vi "captPT01.vi"(6 "Graph in 2":cluster{dbl[], dbl[]}, 8 "error in":errorcluster, 9 "Length 2":i32=250, 11 "ON 2":bool) -> (0 "error out 2":errorcluster caption="error out", 2 "Values 2":cluster{dbl[], dbl[]})   [LabVIEW 2012]
uses:
  GlobalVariables/GantnerParameters.vi
  GlobalVariables/ZeroTimeGraph.vi
  GlobalVariables/CommunicationActivity.vi
  ISMBUS32.DLL
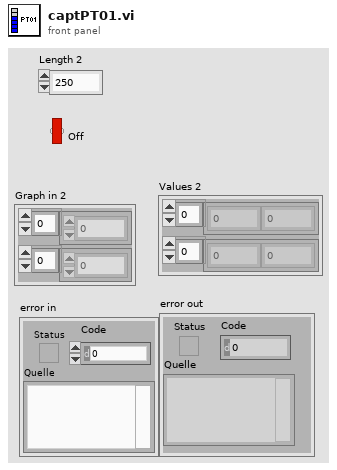
[diagram p1: front panel]
types:
  T1 = typedef "ISMBUS_Module.ctl" = cluster{"ModuleAddress":i32, "ModuleKindIndex":i32, "ModuleKind":string, " Protocol":string, " BaudRate":i32, "CharFormat":string, "BaudRateIndex":i32, "FormatIndex":i32, "ProtocolIndex":i32, "Location":string, "SerialNumber":string, "Vendor":string, "HWRelease":string, "SWRelease":string, "ControllerType":string, "ChannelList":T2[], "ChannelCount":i32, " COM Port":i32}
  T2 = typedef "ISMBUS_Channel.ctl" = cluster{" Description":string, " ChannelKindIndex":i32, "ChannelFormatIndex":i32, " FieldLength":i32, "Precision":i32, "Unit":string, "Mode":i32}
  T3 = cluster{"Module":T1, "PT01 chanel":u32, "Temperature chanel":u32, "HEV01 chanel":u32, "HEV02 chanel":u32, "PressureLimit":dbl}
  T4 = cluster{"KellerActive":bool, "GantnerActive":bool, "BrooksActive":bool}
  T5 = cluster{"KellerActive":bool, bool, "BrooksActive":bool}
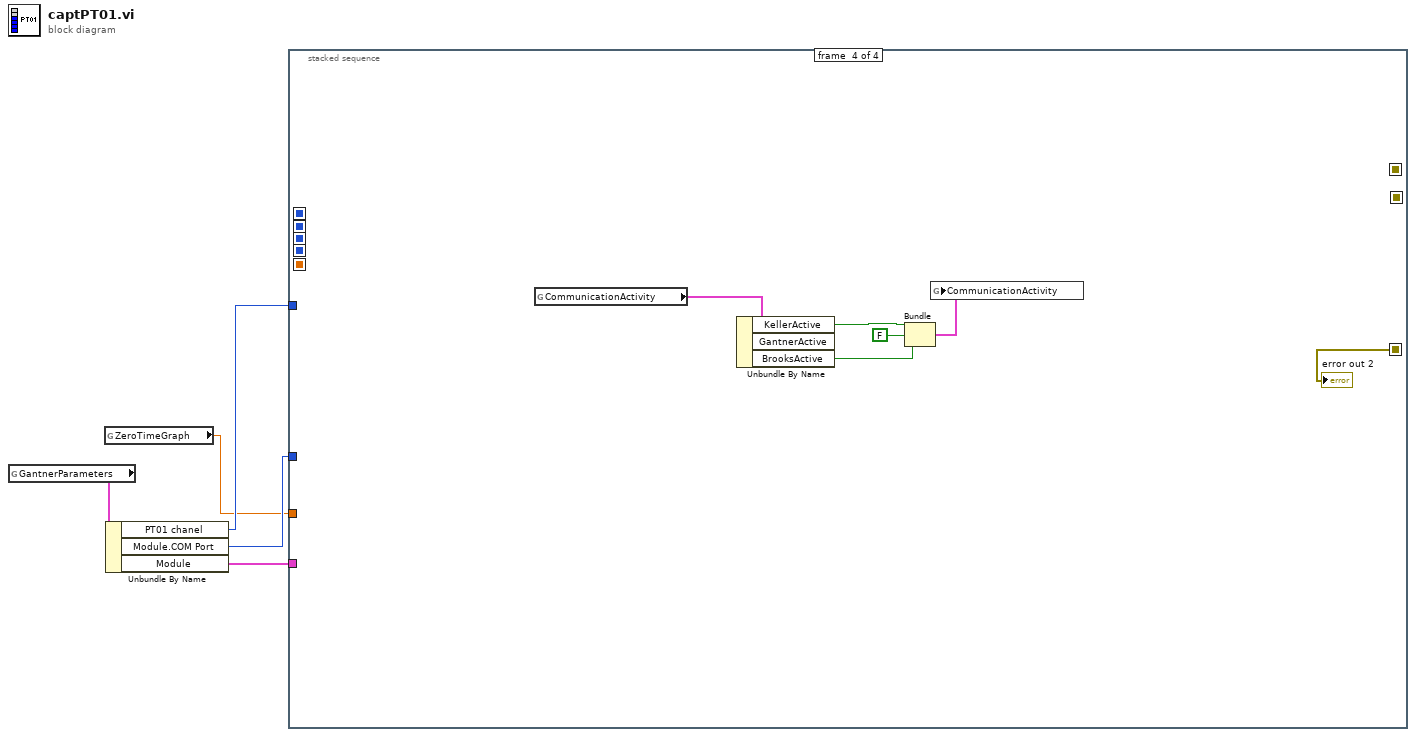
[diagram p0: block diagram]
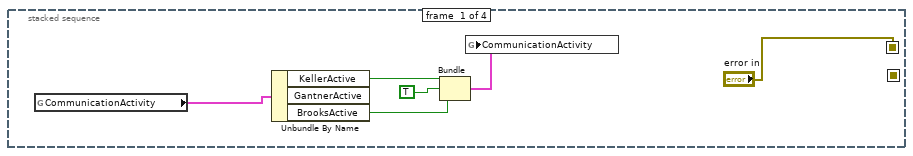
[diagram p2: hidden frame]
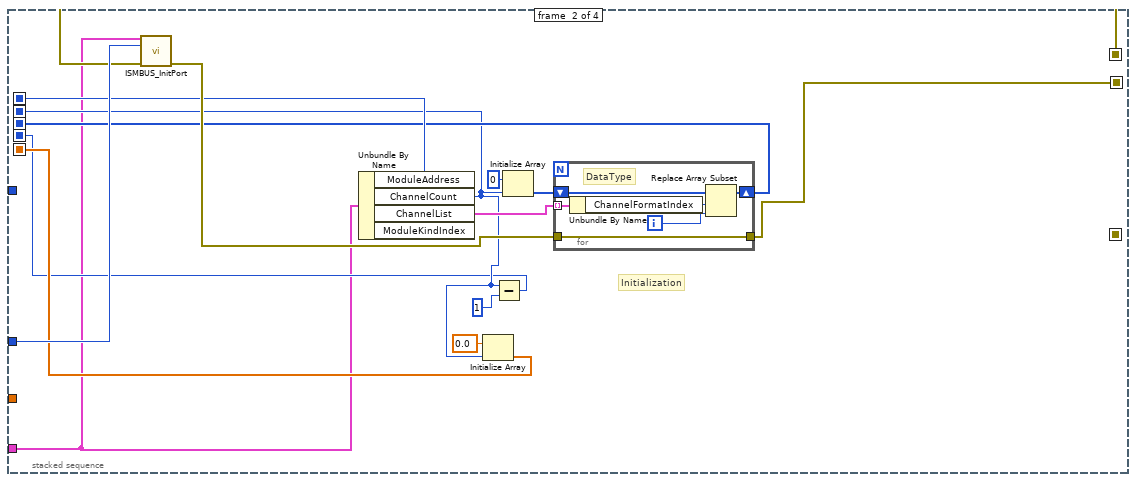
[diagram p3: hidden frame]
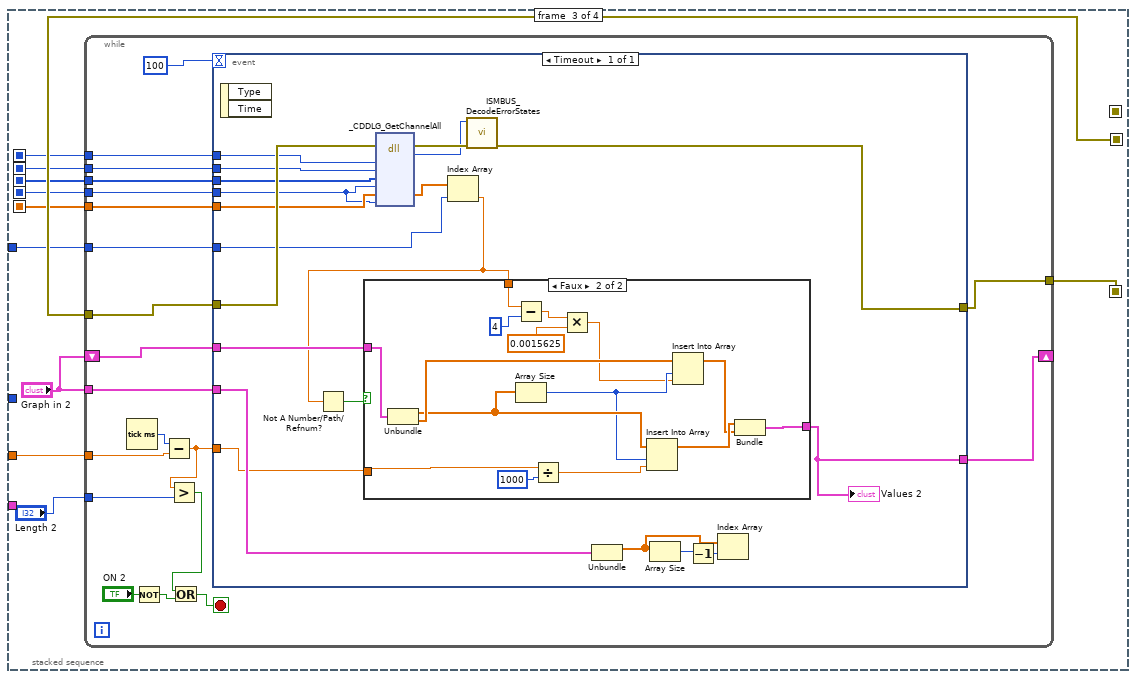
[diagram p4: hidden frame]
diagram:
  n1 = global read "GantnerParameters.vi" "GantnerParameters"() -> (w5:T3)
  n2 = global read "ZeroTimeGraph.vi" "ZeroTimeGraph"() -> (w1:dbl)
  n3 = Unbundle By Name(w5) -> ("PT01 chanel"=w2:u32, "Module.COM Port"=w4:i32, "Module"=w3:T1)
  n4 = stacked-sequence {
    seq-local: ["error in" _ _ _] -> [_ w25 _ _]
    seq-local: [_ _ w41 _] -> [_ _ _ w105]
    seq-local: [_ w18 _ _] -> [_ _ w40 _]
    seq-local: [_ w17 _ _] -> [_ _ w39 _]
    seq-local: [_ w14 _ _] -> [_ _ w38 _]
    seq-local: [_ w16 _ _] -> [_ _ w37 _]
    seq-local: [_ w13 _ _] -> [_ _ w36 _]
    seq-local: [_ w15 _ _] -> [_ _ w35 _]
    tunnel: w4 -> [_ w26 _ _]
    tunnel: w3 -> [_ w12 _ _]
    tunnel: w2 -> [_ _ w34 _]
    tunnel: w1 -> [_ _ w33 _]
    frame #0 {
      n5 = global read "CommunicationActivity.vi" "CommunicationActivity"() -> (w11:T4)
      n6 = Unbundle By Name(w11) -> ("KellerActive"=w7:bool, "BrooksActive"=w9:bool)  [unwired: 1 out]
      n7 = Bundle("KellerActive"=w7, TRUE, "BrooksActive"=w9) -> (w10:T5)  [unwired: 1 in]
      n8 = global write "CommunicationActivity.vi" "CommunicationActivity"(w10) -> ()
    }
    frame #1 {
      # "Initialization"
      n9 = call "ISMBUS_InitPort.vi"("Module"=w12, "ComPort"=w26, "Fehler (Eingang - kein Fehler)"=w25) -> ("Fehler (Ausgang)"=w19:errorcluster)  [unwired: 12 out]
      n10 = Unbundle By Name(w12) -> ("ModuleAddress"=w17:i32, "ChannelCount"=w14:i32, "ChannelList"=w22:T2[])  [unwired: 1 out]
      n11 = Initialize Array(0.0, w14) -> (w15:dbl[])
      n12 = Subtract(x=w14, y=1) -> (x-y=w13:i32)
      n13 = Initialize Array(0 ("Element"), w14) -> (w23:i32[])
      n14 = for {
        tunnel: w22 -> [w31] mode=indexing
        shift-right: [w29] -> w16
        shift-left: w23 -> [w28]
        tunnel: w19 -> [w27]
        tunnel: [w27] -> w18
        i -> [w32]
        # "DataType"
        n15 = Unbundle By Name(w31) -> ("ChannelFormatIndex"=w30:i32)
        n16 = Replace Array Subset(array=w28, new element=w30, index=w32) -> (w29:i32[])
      }
    }
    frame #2 {
      n17 = while {
        tunnel: w40 -> [w62]
        shift-right: [w57] -> _
        shift-left: "Graph in 2" -> [w61]
        tunnel: "Graph in 2" -> [w60]
        tunnel: w33 -> [w58]
        tunnel: "Length 2" -> [w54]
        tunnel: [w50] -> w41
        tunnel: w39 -> [w49]
        tunnel: w38 -> [w48]
        tunnel: w37 -> [w47]
        tunnel: w36 -> [w46]
        tunnel: w35 -> [w45]
        tunnel: w34 -> [w44]
        stop <- w51 stop-if-true
        n18 = Tick Count (ms)() -> (millisecond timer value=w59:u32)
        n19 = Not(x="ON 2") -> (.not. x?=w55:bool)
        n20 = Subtract(x=w59, y=w58) -> (x-y=w53:dbl)
        n21 = Greater?(x=w53, y=w54) -> (0:w52:bool)
        n22 = Or(x=w52, y=w55) -> (x .or. y?=w51:bool)
        n23 = event shown="[0] Timeout" {
          selector: _ -> [_]
          dyn-events: _ -> [_]
          timeout: 100 -> [_]
          tunnel: w62 -> [w75]
          tunnel: [w67] -> w50
          tunnel: w61 -> [w79]
          tunnel: w60 -> [w78]
          tunnel: w53 -> [w77]
          tunnel: [w76] -> w57
          tunnel: w49 -> [w74]
          tunnel: w48 -> [w73]
          tunnel: w47 -> [w72]
          tunnel: w46 -> [w70]
          tunnel: w45 -> [w71]
          tunnel: w44 -> [w65]
          event Timeout {
            n24 = event-data() -> ()  [unwired: 1 in, 2 out]
            n25 = dll-call lib="ISMBUS32.DLL" fn="_CDDLG_GetChannelAll"(error in=w75, "Address"=w74, "NumCh"=w73, "ArrDataTypes"=w72, "ArrDataTypeItemsSub1"=w70, "ArrValues"=w71, "ArrValuesItemsSub1"=w70) -> (error out=w69:errorcluster, w68:i32, "ArrValues"=w66:dbl[])  [unwired: 7 in, 1 out]
            n26 = Index Array(array=w66, index=w65) -> (element=w64:dbl)
            n27 = Not A Number/Path/Refnum?(number/path/refnum=w64) -> (NaN/Path/Refnum?=w80:bool)
            n28 = case shown="Faux" w80 {
              tunnel: w77 -> [_ w99]
              tunnel: w64 -> [_ w90]
              tunnel: w79 -> [w84 w97]
              tunnel: [w84 w96] -> w76
              frame True {
              }
              frame False {
                n29 = Unbundle(w97) -> (w92:dbl[], w93:dbl[])
                n30 = Subtract(x=w90, y=4) -> (x-y=w88:dbl)
                n31 = Array Size(array=w92) -> (size(s)=w91:i32)
                n32 = Divide(x=w99, y=1000) -> (x/y=w85:dbl)
                n33 = Multiply(x=w88, y=0.0015625) -> (x*y=w86:dbl)
                n34 = Insert Into Array(array=w92, index=w91, new element=w85) -> (w95:dbl[])
                n35 = Insert Into Array(array=w93, index=w91, new element=w86) -> (w94:dbl[])
                n36 = Bundle(w95, w94) -> (w96:cluster{dbl[], dbl[]})  [unwired: 1 in]
              }
            }
            "Values 2" <- w76
            n37 = call "ISMBUS_DecodeErrorStates.vi"("Fehler (Eingang - kein Fehler)"=w69, "ISMBUS_Error State"=w68) -> ("Fehler (Ausgang)"=w67:errorcluster)  [unwired: 1 in, 8 out]
            n38 = Unbundle(w78) -> (w81:dbl[])  [unwired: 1 out]
            n39 = Array Size(array=w81) -> (size(s)=w83:i32)
            n40 = Decrement(x=w83) -> (x-1=w82:i32)
            n41 = Index Array(array=w81, index=w82) -> ()  [unwired: 1 out]
          }
        }
      }
    }
    frame #3 {
      n42 = global read "CommunicationActivity.vi" "CommunicationActivity"() -> (w104:T4)
      n43 = Unbundle By Name(w104) -> ("KellerActive"=w101:bool, "BrooksActive"=w102:bool)  [unwired: 1 out]
      n44 = Bundle("KellerActive"=w101, FALSE, "BrooksActive"=w102) -> (w103:T5)  [unwired: 1 in]
      n45 = global write "CommunicationActivity.vi" "CommunicationActivity"(w103) -> ()
      "error out 2" <- w105
    }
  }
